vi "Delay-processing.vi"(8 "error in":errorcluster, 10 "UI ref. in":refnum<data-value>, 11 "Data ref. in":refnum<data-value>) -> (0 "error IO":errorcluster, 2 "UI ref.":refnum<data-value>, 3 "Data ref.":refnum<data-value>)   [LabVIEW 2013, in "CameraVision.lvlib" / "CV-Main.lvclass"]
doc: "This function increases the layer/iteration number by one (+1)."
uses:
  CV-Main.lvclass
  UI/CV-UI.lvclass
  UI/CV-UI.lvclass/CV-UI.ctl
  CV-Main.lvclass/CV-Main.ctl
  Acquisition/CV-Acquisition.lvclass/CV-Acquisition.ctl
  UI/Notifier-with-memory-boolean.vi
  UI/Read Acquisition.vi
  Read Acquis params.vi
  Acquisition/Read Acquisition mode.vi
  Acquisition/CV-Acquisition.lvclass
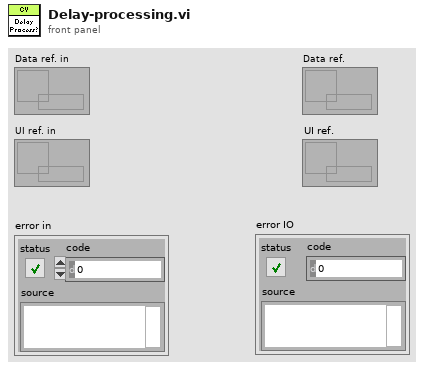
[diagram p1: front panel]
types:
  T1 = enum16{"Continuous", "Continuous batch", "Single batch", "Single batch -delayed"}
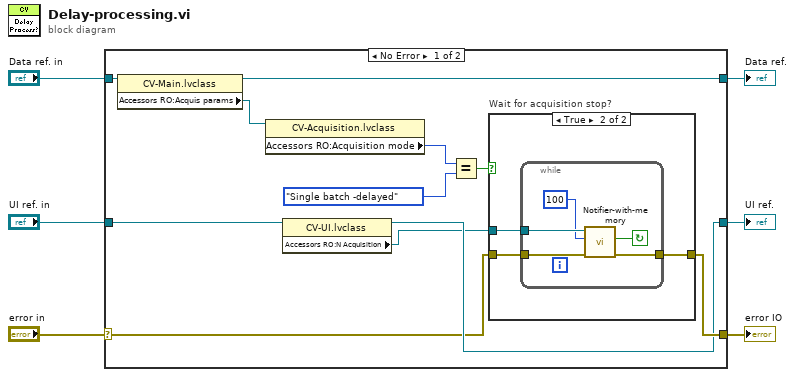
[diagram p0: block diagram]
diagram:
  n1 = case shown="No Error" "error in" {
    selector: "error in" -> [w7 w29]
    tunnel: [w11 w29] -> w5
    tunnel: "Data ref. in" -> [w17 w28]
    tunnel: [w16 w28] -> w3
    tunnel: "UI ref. in" -> [w12 w27]
    tunnel: [w9 w27] -> w1
    frame No Error {
      n2 = property class="CV-Main.lvclass"(reference=w17) -> (reference out=w16:refnum<data-value>, "Accessors RO:Acquis params"=w10:refnum<data-value>)  [unwired: 1 in, 1 out]
      n3 = property class="CV-Acquisition.lvclass"(reference=w10) -> ("Accessors RO:Acquisition mode"=w15:T1)  [unwired: 1 in, 2 out]
      n4 = property class="CV-UI.lvclass"(reference=w12) -> (reference out=w9:refnum<data-value>, "Accessors RO:N Acquisition"=w8:refnum<notifier>)  [unwired: 1 in, 1 out]
      n5 = Equal?(x=w15, y=T1."Single batch -delayed") -> (x = y?=w13:bool)
      n6 = case "Wait for acquisition stop?" shown="True" w13 {
        tunnel: w8 -> [_ w21]
        tunnel: w7 -> [w18 w20]
        tunnel: [w18 w19] -> w11
        frame False {
        }
        frame True {
          n7 = while {
            tunnel: w21 -> [w26]
            tunnel: w20 -> [w25]
            tunnel: [w24] -> w19
            stop <- w23 continue-if-true
            n8 = call-poly "Notifier-with-memory.vi"("error in"=w25, "Timeout [ms]"=100 ("milliseconds to wait"), "Notifier in"=w26) -> ("error IO"=w24:errorcluster, "Notification"=w23:bool)  [unwired: 7 in]
          }
        }
      }
    }
    frame Error {
    }
  }
  "error IO" <- w5
  "Data ref." <- w3
  "UI ref." <- w1
